vi "extract_central.vi"(8 "error in (no error)":errorcluster, 9 "size":dbl=2.0, 10 "Image Dst":T1, 11 "Image":T1) -> (0 "error out":errorcluster, 3 "Image Dst Out":T1)   [LabVIEW 2016]
doc: "Extracts central square from image of specified size."
uses:
  <vilib>/vision/Image Controls.llb/IMAQ Image.ctl
  <vilib>/vision/NI_Vision_Development_Module.lvlib
panel:
  out "co-ordinates":dbl[](array[numeric])
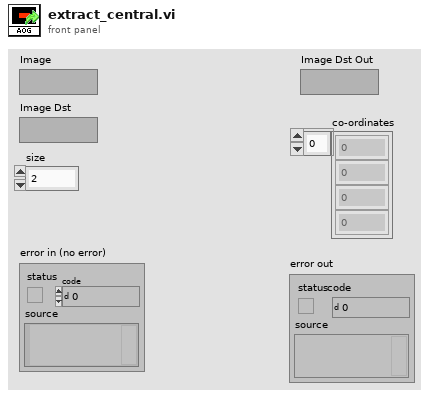
[diagram p1: front panel]
types:
  T1 = typedef "IMAQ Image.ctl" = refnum<image>
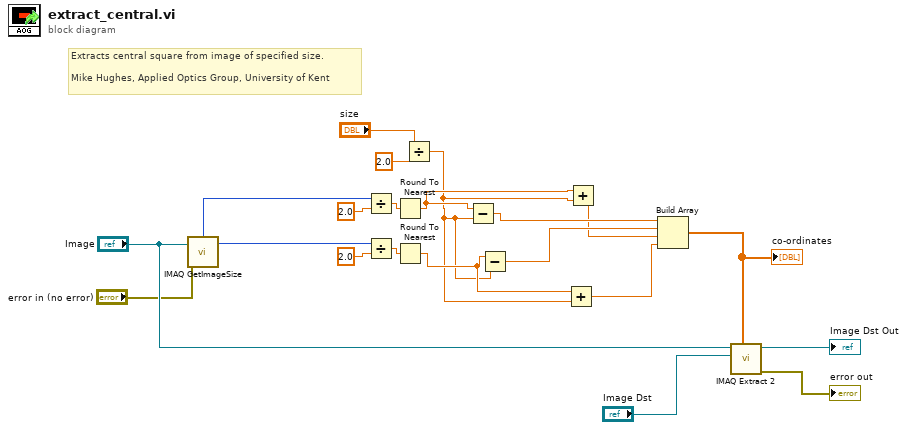
[diagram p0: block diagram]
diagram:
  # "Extracts central square from image of specified size.\n\nMike Hughes, Applied Optics Group, University of Kent"
  n1 = call "IMAQ GetImageSize"("Image"="Image", "error in (no error)"="error in (no error)") -> ("Y Resolution"=w15:i32, "X Resolution"=w19:i32)  [unwired: 2 in, 1 out]
  n2 = Divide(x=w19, y=2.0) -> (x/y=w18:dbl)
  n3 = Divide(x=w15, y=2.0) -> (x/y=w16:dbl)
  n4 = Round To Nearest(number=w18) -> (nearest integer value=w3:dbl)
  n5 = Round To Nearest(number=w16) -> (nearest integer value=w2:dbl)
  n6 = Divide(x="size", y=2.0) -> (x/y=w1:dbl)
  n7 = Subtract(x=w3, y=w1) -> (x-y=w14:dbl)
  n8 = Subtract(x=w2, y=w1) -> (x-y=w13:dbl)
  n9 = Add(x=w2, y=w1) -> (x+y=w11:dbl)
  n10 = Add(x=w3, y=w1) -> (x+y=w12:dbl)
  n11 = Build Array(w14, w13, w12, w11) -> (w10:dbl[])
  "co-ordinates" <- w10
  n12 = call "IMAQ Extract 2"("Optional Rectangle"=w10, "Image Dst"="Image Dst", "Image Src"="Image") -> ("error out"=→"error out":errorcluster, "Image Dst Out"=→"Image Dst Out":T1)  [unwired: 7 in]
